vi "核查数据时间戳转换 (子VI).vi"(10 "枚举":enum16{"零点跨度", "标样核查"}(ring), 11 "核查索引":string[](array[string])) -> (3 "数组":string[](array[string]))   [LabVIEW 2016, in "数据传输系统.lvlib"]
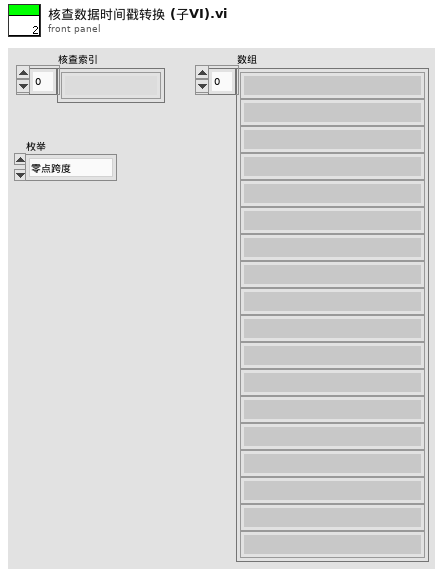
[diagram p1: front panel]
types:
  T1 = typedef "LVDateTimeRec.ctl" = cluster{"秒数的小数部分":dbl, "秒":i32, "分":i32, "时":i32, "日":i32, "月":i32, "年":i32, "天数（周）":i32, "天数（年）":i32, "DST":i32}
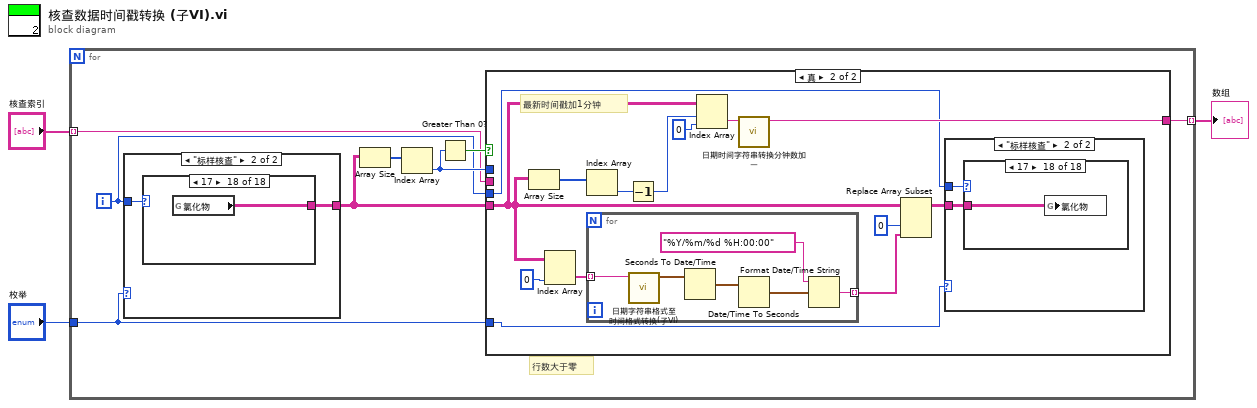
[diagram p0: block diagram]
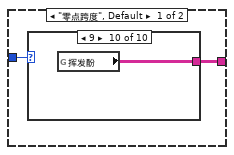
[diagram p2: hidden frame]
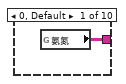
[diagram p3: hidden frame]
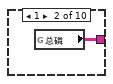
[diagram p4: hidden frame]
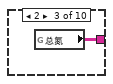
[diagram p5: hidden frame]
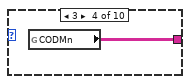
[diagram p6: hidden frame]
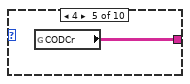
[diagram p7: hidden frame]
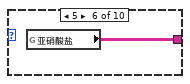
[diagram p8: hidden frame]
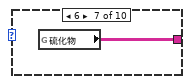
[diagram p9: hidden frame]
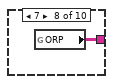
[diagram p10: hidden frame]
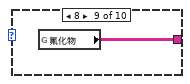
[diagram p11: hidden frame]
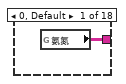
[diagram p12: hidden frame]
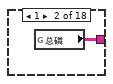
[diagram p13: hidden frame]
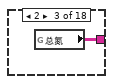
[diagram p14: hidden frame]
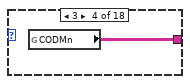
[diagram p15: hidden frame]
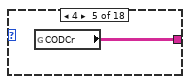
[diagram p16: hidden frame]
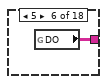
[diagram p17: hidden frame]
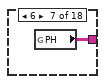
[diagram p18: hidden frame]
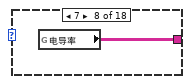
[diagram p19: hidden frame]
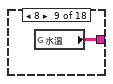
[diagram p20: hidden frame]
diagram:
  n1 = for {
    tunnel: [w8] -> w3 mode=indexing
    tunnel: "核查索引" -> [w7] mode=indexing
    tunnel: "枚举" -> [w4]
    i -> [w6]
    # "行数大于零"
    n2 = case shown="\"标样核查\"" w4 {
      tunnel: w6 -> [w12 w25]
      tunnel: [w13 w24] -> w5
      frame "零点跨度", Default {
        n3 = case shown="9" w12 {
          tunnel: [w14 w15 w16 w17 w18 w19 w20 w21 w22 w23] -> w13
          frame 0, Default {
            n4 = global read "全局 所有参数.vi" "氨氮"() -> (w14:string[][])
          }
          frame 1 {
            n5 = global read "全局 所有参数.vi" "总磷"() -> (w15:string[][])
          }
          frame 2 {
            n6 = global read "全局 所有参数.vi" "总氮"() -> (w16:string[][])
          }
          frame 3 {
            n7 = global read "全局 所有参数.vi" "CODMn"() -> (w17:string[][])
          }
          frame 4 {
            n8 = global read "全局 所有参数.vi" "CODCr"() -> (w18:string[][])
          }
          frame 5 {
            n9 = global read "全局 所有参数.vi" "亚硝酸盐"() -> (w19:string[][])
          }
          frame 6 {
            n10 = global read "全局 所有参数.vi" "硫化物"() -> (w20:string[][])
          }
          frame 7 {
            n11 = global read "全局 所有参数.vi" "ORP"() -> (w21:string[][])
          }
          frame 8 {
            n12 = global read "全局 所有参数.vi" "氟化物"() -> (w22:string[][])
          }
          frame 9 {
            n13 = global read "全局 所有参数.vi" "挥发酚"() -> (w23:string[][])
          }
        }
      }
      frame "标样核查" {
        n14 = case shown="17" w25 {
          tunnel: [w26 w27 w28 w29 w30 w31 w32 w33 w34 w35 w36 w37 w38 w39 w40 w41 w42 w43] -> w24
          frame 0, Default {
            n15 = global read "全局 所有参数.vi" "氨氮"() -> (w26:string[][])
          }
          frame 1 {
            n16 = global read "全局 所有参数.vi" "总磷"() -> (w27:string[][])
          }
          frame 2 {
            n17 = global read "全局 所有参数.vi" "总氮"() -> (w28:string[][])
          }
          frame 3 {
            n18 = global read "全局 所有参数.vi" "CODMn"() -> (w29:string[][])
          }
          frame 4 {
            n19 = global read "全局 所有参数.vi" "CODCr"() -> (w30:string[][])
          }
          frame 5 {
            n20 = global read "全局 所有参数.vi" "DO"() -> (w31:string[][])
          }
          frame 6 {
            n21 = global read "全局 所有参数.vi" "PH"() -> (w32:string[][])
          }
          frame 7 {
            n22 = global read "全局 所有参数.vi" "电导率"() -> (w33:string[][])
          }
          frame 8 {
            n23 = global read "全局 所有参数.vi" "水温"() -> (w34:string[][])
          }
          frame 9 {
            n24 = global read "全局 所有参数.vi" "浊度"() -> (w35:string[][])
          }
          frame 10 {
            n25 = global read "全局 所有参数.vi" "叶绿素"() -> (w36:string[][])
          }
          frame 11 {
            n26 = global read "全局 所有参数.vi" "藻密度"() -> (w37:string[][])
          }
          frame 12 {
            n27 = global read "全局 所有参数.vi" "亚硝酸盐"() -> (w38:string[][])
          }
          frame 13 {
            n28 = global read "全局 所有参数.vi" "硫化物"() -> (w39:string[][])
          }
          frame 14 {
            n29 = global read "全局 所有参数.vi" "ORP"() -> (w40:string[][])
          }
          frame 15 {
            n30 = global read "全局 所有参数.vi" "氟化物"() -> (w41:string[][])
          }
          frame 16 {
            n31 = global read "全局 所有参数.vi" "挥发酚"() -> (w42:string[][])
          }
          frame 17 {
            n32 = global read "全局 所有参数.vi" "氯化物"() -> (w43:string[][])
          }
        }
      }
    }
    n33 = Array Size(array=w5) -> (size(s)=w10:i32[])
    n34 = Index Array(array=w10) -> (element=w9:i32)  [unwired: 1 in]
    n35 = Greater Than 0?(x=w9) -> (x > 0?=w11:bool)
    n36 = case shown="真" w11 {
      tunnel: w9 -> [_ _]
      tunnel: w5 -> [_ w50]
      tunnel: [w44 w54] -> w8
      tunnel: w7 -> [w44 _]
      tunnel: w6 -> [_ w46]
      tunnel: w4 -> [_ w45]
      frame False {
      }
      frame True {
        # "最新时间戳加1分钟"
        n37 = Array Size(array=w50) -> (size(s)=w58:i32[])
        n38 = Index Array(array=w50, index (col)=0 ("禁用的索引 (列)")) -> (element=w51:string[])  [unwired: 1 in]
        n39 = Index Array(array=w58) -> (element=w57:i32)  [unwired: 1 in]
        n40 = for {
          tunnel: w51 -> [w92] mode=indexing
          tunnel: [w91] -> w48 mode=indexing
          n41 = call "日期字符串格式至时间格式转换(子VI).vi"("data[0]"=w92) -> ("time stamp"=w94:timestamp)  [unwired: 10 in]
          n42 = Seconds To Date/Time(time stamp (now)=w94) -> (date time rec=w93:T1)  [unwired: 1 in]
          n43 = Date/Time To Seconds(2:w93) -> (0:w95:timestamp)  [unwired: 1 in]
          n44 = Format Date/Time String(time format string (%c)="%Y/%m/%d %H:00:00" ("时间格式字符串(%c)"), seconds (now)=w95) -> (date/time string=w91:string)  [unwired: 1 in]
        }
        n45 = Decrement(x=w57) -> (x-1=w56:i32)
        n46 = Index Array(array=w50, index (row)=w56, index (col)=0 ("禁用的索引 (列)")) -> (element=w53:string)
        n47 = call "日期时间字符串转换分钟数加一.vi"("data[0]"=w53) -> ("日期/时间字符串"=w54:string)  [unwired: 10 in]
        n48 = Replace Array Subset(array=w50, new element=w48, index (col)=0 ("禁用的索引 (列)")) -> (w47:string[][])  [unwired: 1 in]
        n49 = case shown="\"标样核查\"" w45 {
          tunnel: w46 -> [w59 w72]
          tunnel: w47 -> [w60 w71]
          frame "零点跨度", Default {
            n50 = case shown="9" w59 {
              tunnel: w60 -> [w61 w62 w63 w64 w65 w66 w67 w68 w69 w70]
              frame 0, Default {
                n51 = global write "全局 所有参数.vi" "氨氮"(w61) -> ()
              }
              frame 1 {
                n52 = global write "全局 所有参数.vi" "总磷"(w62) -> ()
              }
              frame 2 {
                n53 = global write "全局 所有参数.vi" "总氮"(w63) -> ()
              }
              frame 3 {
                n54 = global write "全局 所有参数.vi" "CODMn"(w64) -> ()
              }
              frame 4 {
                n55 = global write "全局 所有参数.vi" "CODCr"(w65) -> ()
              }
              frame 5 {
                n56 = global write "全局 所有参数.vi" "亚硝酸盐"(w66) -> ()
              }
              frame 6 {
                n57 = global write "全局 所有参数.vi" "硫化物"(w67) -> ()
              }
              frame 7 {
                n58 = global write "全局 所有参数.vi" "ORP"(w68) -> ()
              }
              frame 8 {
                n59 = global write "全局 所有参数.vi" "氟化物"(w69) -> ()
              }
              frame 9 {
                n60 = global write "全局 所有参数.vi" "挥发酚"(w70) -> ()
              }
            }
          }
          frame "标样核查" {
            n61 = case shown="17" w72 {
              tunnel: w71 -> [w73 w74 w75 w76 w77 w78 w79 w80 w81 w82 w83 w84 w85 w86 w87 w88 w89 w90]
              frame 0, Default {
                n62 = global write "全局 所有参数.vi" "氨氮"(w73) -> ()
              }
              frame 1 {
                n63 = global write "全局 所有参数.vi" "总磷"(w74) -> ()
              }
              frame 2 {
                n64 = global write "全局 所有参数.vi" "总氮"(w75) -> ()
              }
              frame 3 {
                n65 = global write "全局 所有参数.vi" "CODMn"(w76) -> ()
              }
              frame 4 {
                n66 = global write "全局 所有参数.vi" "CODCr"(w77) -> ()
              }
              frame 5 {
                n67 = global write "全局 所有参数.vi" "DO"(w78) -> ()
              }
              frame 6 {
                n68 = global write "全局 所有参数.vi" "PH"(w79) -> ()
              }
              frame 7 {
                n69 = global write "全局 所有参数.vi" "电导率"(w80) -> ()
              }
              frame 8 {
                n70 = global write "全局 所有参数.vi" "水温"(w81) -> ()
              }
              frame 9 {
                n71 = global write "全局 所有参数.vi" "浊度"(w82) -> ()
              }
              frame 10 {
                n72 = global write "全局 所有参数.vi" "叶绿素"(w83) -> ()
              }
              frame 11 {
                n73 = global write "全局 所有参数.vi" "藻密度"(w84) -> ()
              }
              frame 12 {
                n74 = global write "全局 所有参数.vi" "亚硝酸盐"(w85) -> ()
              }
              frame 13 {
                n75 = global write "全局 所有参数.vi" "硫化物"(w86) -> ()
              }
              frame 14 {
                n76 = global write "全局 所有参数.vi" "ORP"(w87) -> ()
              }
              frame 15 {
                n77 = global write "全局 所有参数.vi" "氟化物"(w88) -> ()
              }
              frame 16 {
                n78 = global write "全局 所有参数.vi" "挥发酚"(w89) -> ()
              }
              frame 17 {
                n79 = global write "全局 所有参数.vi" "氯化物"(w90) -> ()
              }
            }
          }
        }
      }
    }
  }
  "数组" <- w3
